vi "Simpson's Rule.vi"(9 "delta_x":dbl, 10 "Array":dbl[](array[numeric])) -> (2 "Value of Integral":dbl)   [LabVIEW 2017]
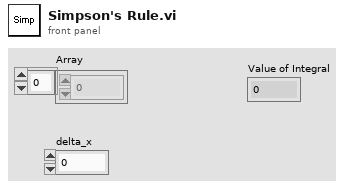
[diagram p1: front panel]
types:
  T1 = cluster{"Number of Partial Sums":i32, "Odd?":bool}
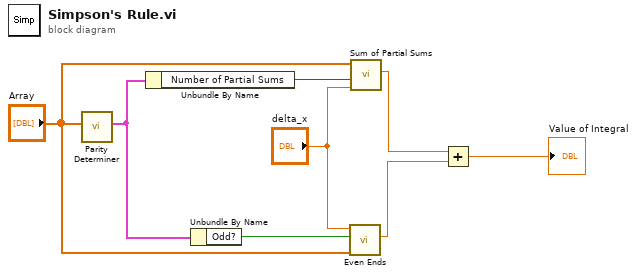
[diagram p0: block diagram]
diagram:
  n1 = call "Parity Determiner.vi"("Array"="Array") -> ("Output Cluster"=w5:T1)  [unwired: 10 in]
  n2 = Unbundle By Name(w5) -> ("Number of Partial Sums"=w8:i32)
  n3 = Unbundle By Name(w5) -> ("Odd?"=w4:bool)
  n4 = call "Even Ends.vi"("Array"="Array", "Odd?"=w4, "delta_x"="delta_x") -> ("Trap Value"=w2:dbl)  [unwired: 8 in]
  n5 = call "Sum of Partial Sums.vi"("delta_x"="delta_x", "Number of Partial Sum"=w8, "Array"="Array") -> ("Simp Value"=w3:dbl)  [unwired: 8 in]
  n6 = Add(x=w3, y=w2) -> (x+y=→"Value of Integral":dbl)
